vi "ConsumerProcess.vi"(7 "SubQueueIN":refnum<queue>, 8 "error in (no error)":errorcluster, 9 "Command":T1, 10 "MainQueueIN":refnum<queue>, 11 "Data Value Reference IN":refnum<data-value>) -> (0 "error out":errorcluster, 3 "Data Value Reference out":refnum<data-value>)   [LabVIEW 2013]
uses:
  Control/SystemData.ctl
  Control/SignalType.ctl
  Control/SystemCommand.ctl
  Control/SubDaqCommand.ctl
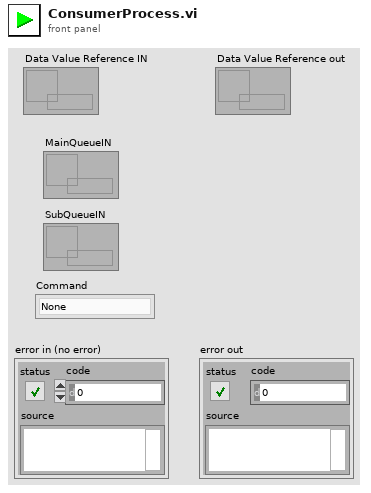
[diagram p1: front panel]
types:
  T1 = typedef "SystemCommand.ctl" = enum16{"None", "Init", "Close", "ShowNumeric", "ShowString", "ShowBool", "SquareNumeric", "ReverseString", "InvertBool", "FFT"}
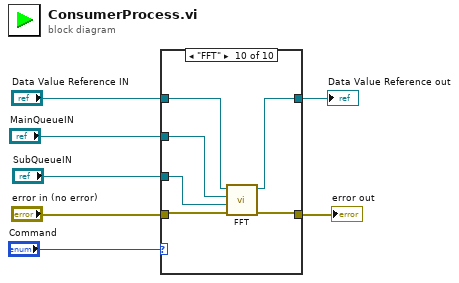
[diagram p0: block diagram]
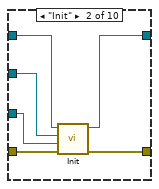
[diagram p3: hidden frame]
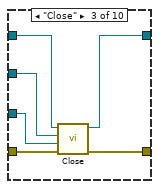
[diagram p4: hidden frame]
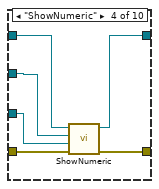
[diagram p5: hidden frame]
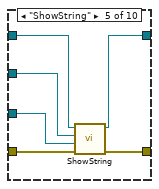
[diagram p6: hidden frame]
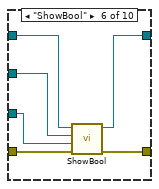
[diagram p7: hidden frame]
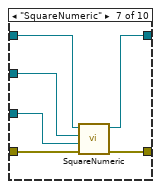
[diagram p8: hidden frame]
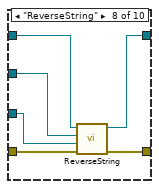
[diagram p9: hidden frame]
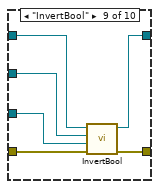
[diagram p10: hidden frame]
diagram:
  n1 = case shown="\"FFT\"" "Command" {
    tunnel: "Data Value Reference IN" -> [w9 w12 w18 w25 w33 w36 w45 w51 w53 w60]
    tunnel: [w9 w11 w17 w24 w29 w37 w41 w47 w57 w59] -> w6
    tunnel: "error in (no error)" -> [w8 w14 w20 w27 w31 w38 w43 w49 w56 w63]
    tunnel: [w8 w13 w19 w23 w30 w39 w42 w48 w55 w58] -> w7
    tunnel: "MainQueueIN" -> [_ w15 w21 w26 w32 w35 w44 w50 w54 w61]
    tunnel: "SubQueueIN" -> [_ w10 w16 w22 w28 w34 w40 w46 w52 w62]
    frame Default {
    }
    frame "Init" {
      n2 = call "Init.vi"("error in (no error)"=w14, "SubQueueIN"=w10, "MainQueueIN"=w15, "Data Value Reference IN"=w12) -> ("error out"=w13:errorcluster, "Data Value Reference out"=w11:refnum<data-value>)  [unwired: 6 in]
    }
    frame "Close" {
      n3 = call "Close.vi"("error in (no error)"=w20, "SubQueueIN"=w16, "MainQueueIN"=w21, "Data Value Reference IN"=w18) -> ("error out"=w19:errorcluster, "Data Value Reference out"=w17:refnum<data-value>)  [unwired: 6 in]
    }
    frame "ShowNumeric" {
      n4 = call "ShowNumeric.vi"("error in (no error)"=w27, "SubQueueIN"=w22, "MainQueueIN"=w26, "Data Value Reference IN"=w25) -> ("error out"=w23:errorcluster, "Data Value Reference out"=w24:refnum<data-value>)  [unwired: 6 in]
    }
    frame "ShowString" {
      n5 = call "ShowString.vi"("error in (no error)"=w31, "SubQueueIN"=w28, "MainQueueIN"=w32, "Data Value Reference out"=w33) -> ("error out"=w30:errorcluster, "Data Value Reference out"=w29:refnum<data-value>)  [unwired: 6 in]
    }
    frame "ShowBool" {
      n6 = call "ShowBool.vi"("error in (no error)"=w38, "SubQueueIN"=w34, "MainQueueIN"=w35, "Data Value Reference IN"=w36) -> ("error out"=w39:errorcluster, "Data Value Reference out"=w37:refnum<data-value>)  [unwired: 6 in]
    }
    frame "SquareNumeric" {
      n7 = call "SquareNumeric.vi"("error in (no error)"=w43, "SubQueueIN"=w40, "MainQueueIN"=w44, "Data Value Reference IN"=w45) -> ("error out"=w42:errorcluster, "Data Value Reference out"=w41:refnum<data-value>)  [unwired: 6 in]
    }
    frame "ReverseString" {
      n8 = call "ReverseString.vi"("error in (no error)"=w49, "SubQueueIN"=w46, "MainQueueIN"=w50, "Data Value Reference IN"=w51) -> ("error out"=w48:errorcluster, "Data Value Reference out"=w47:refnum<data-value>)  [unwired: 6 in]
    }
    frame "InvertBool" {
      n9 = call "InvertBool.vi"("error in (no error)"=w56, "SubQueueIN"=w52, "MainQueueIN"=w54, "Data Value Reference IN"=w53) -> ("error out"=w55:errorcluster, "Data Value Reference out"=w57:refnum<data-value>)  [unwired: 6 in]
    }
    frame "FFT" {
      n10 = call "FFT.vi"("error in (no error)"=w63, "SubQueueIN"=w62, "MainQueueIN"=w61, "Data Value Reference IN"=w60) -> ("error out"=w58:errorcluster, "Data Value Reference out"=w59:refnum<data-value>)  [unwired: 6 in]
    }
  }
  "error out" <- w7
  "Data Value Reference out" <- w6
